vi "Test CN79000 Code.vi"() -> ()   [LabVIEW 2014]
uses:
  CN79000.lvclass
  <vilib>/addons/_NISVFA/_Shared subVIs/Data Objects/Data/Data.lvclass
panel:
  in  "Boolean":bool
  out "DataArray":refnum<class "Data.lvclass">[](array[class])
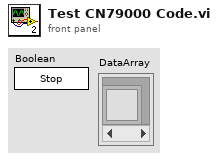
[diagram p1: front panel]
types:
  T1 = cluster{"baud rate (9600)":u32, "data bits (8)":u16, "stop bits (10: 1 bit)":u16, "termination char\n(0xA = '\\n' = LF) ":u8, "parity (0:none)":enum16{"None", "Odd", "Even", "Mark", "Space"}, "timeout (10sec)":u32, "Enable Termination\nChar (T)":bool, "flow control (0:none)":u16}
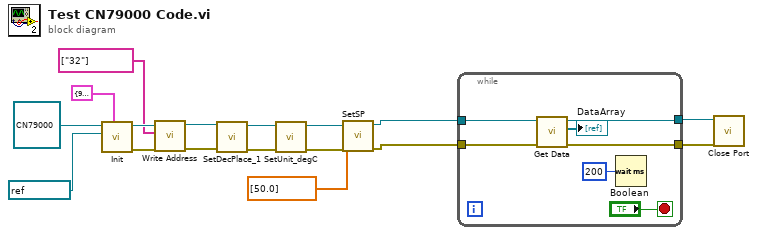
[diagram p0: block diagram]
diagram:
  n1 = call-dynamic "Init.vi"("PortCfg"=T1 {"baud rate (9600)"=9600, "data bits (8)"=8, "stop bits (10: 1 bit)"=10, "termination char\n(0xA = '\\n' = LF) "=10, "parity (0:none)"=enum."None", "timeout (10sec)"=10000, "Enable Termination\nChar (T)"=TRUE, "flow control (0:none)"=0}, "Port"=refnum<visa-resource-name> "COM5", "Serial IO in"=refnum<class "CN79000.lvclass"> refnum ("CN79000.lvclass")) -> ("error out"=w9:errorcluster, "Serial IO out"=w10:refnum<class "CN79000.lvclass">)  [unwired: 7 in]
  n2 = call "Write Address.vi"("error in"=w9, "Address"=string[] ["32"], "CN79000 in"=w10) -> ("error out"=w7:errorcluster, "CN79000 out"=w8:refnum<class "CN79000.lvclass">)  [unwired: 7 in]
  n3 = call "SetDecPlace_1.vi"("error in"=w7, "CN79000 in"=w8) -> ("error out"=w15:errorcluster, "CN79000 out"=w16:refnum<class "CN79000.lvclass">)  [unwired: 8 in]
  n4 = call "SetUnit_degC.vi"("error in"=w15, "CN79000 in"=w16) -> ("error out"=w11:errorcluster, "CN79000 out"=w12:refnum<class "CN79000.lvclass">)  [unwired: 8 in]
  n5 = call "SetSP.vi"("error in (no error)"=w11, "ctlSP"=dbl[] [50.0], "CN79000 in"=w12) -> ("error out"=w3:errorcluster, "CN79000 out"=w4:refnum<class "CN79000.lvclass">)  [unwired: 7 in]
  n6 = while {
    tunnel: w4 -> [w24]
    tunnel: w3 -> [w23]
    tunnel: [w22] -> w2
    tunnel: [w21] -> w1
    stop <- "Boolean" stop-if-true
    n7 = call-dynamic "Get Data.vi"("error in (no error)"=w23, "CN79000 in"=w24) -> ("error out"=w21:errorcluster, "DataArray"=→"DataArray":refnum<class "Data.lvclass">[], "CN79000 out"=w22:refnum<class "CN79000.lvclass">)  [unwired: 7 in]
    n8 = Wait (ms)(milliseconds to wait=u32 200) -> ()  [unwired: 1 out]
  }
  n9 = call-dynamic "Close Port.vi"("error in (no error)"=w1, "Serial IO in"=w2) -> ()  [unwired: 8 in, 2 out]
